vi "程序调试.vi"() -> ()   [LabVIEW 2010]
panel:
  out "颜色盒":u32(colorbox)
  in  "停止":bool
  in  "y":dbl
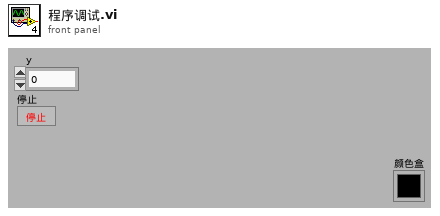
[diagram p1: front panel]
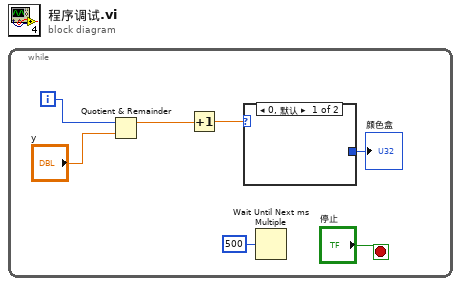
[diagram p0: block diagram]
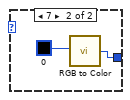
[diagram p2: hidden frame]
diagram:
  n1 = while {
    i -> [w7]
    stop <- "停止" stop-if-true
    n2 = Quotient & Remainder(x=w7, y="y") -> (x-y*floor(x/y)=w5:dbl)  [unwired: 1 out]
    n3 = Increment(x=w5) -> (x+1=w2:dbl)
    n4 = case shown="0, 默认" w2 {
      tunnel: [_ w8] -> w1
      frame 0, Default {
      }
      frame 7 {
        n5 = call <vilib>:"RGB to Color.vi"("G"=u32 0 ("颜色盒")) -> ("Color"=w8:u32)  [unwired: 2 in]
      }
    }
    "颜色盒" <- w1
    n6 = Wait Until Next ms Multiple(millisecond multiple=u32 500 ("毫秒倍数")) -> ()  [unwired: 1 out]
  }
